vi "String to AUX device cluster.vi"(11 "AUX Device Details":string="GFSF:50:SPD:2:MAN:HVER:1:FVER:0.1:SERL:1837600001:MAN:GMIN:5:TES:3:SIG:OPEN:50.6:STEP:7:SIG:GEAR:6:TVES:19:AUX") -> (3 "Auxiliary Device":T1 {"Signals"."% Open" min=0.0 max=100.0 step=0.1 format="%.4f"; "Signals"."Position" max=20.0 step=1.0 format="%.4f"; "Speed" max=7 step=1; "Gear" max=7 step=1; "Temp V Err" min=0.0 max=20.0 step=0.1; "Temp Err" min=0.0 max=20.0 step=0.1; "Scaling Factor" min=0.0 max=99.0 step=0.1; "Min Flow" min=0.0 max=20.0 step=0.1})   [LabVIEW 2019, in "Mercury iXX.lvlib" / "Auxiliary.lvlib"]
uses:
  Auxiliary.lvlib
  Controls/AUX Device (Read).ctl
  Controls/Manufacturing Data.ctl
  Controls/AUX Signals (Read).ctl
  Mercury iXX.lvlib
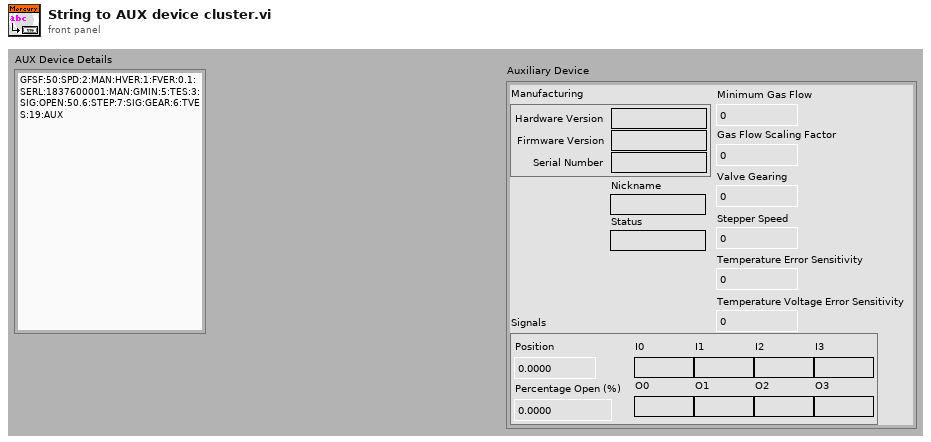
[diagram p1: front panel]
types:
  T1 = typedef "Mercury iXX.lvlib/Auxiliary.lvlib/AUX Device (Read).ctl" = cluster{"Manufacturing":T2, "Min Flow":dbl, "Scaling Factor":dbl, "Temp Err":dbl, "Temp V Err":dbl, "Gear":u32, "Speed":u32, "Signals":T3, "Nickname":string, "Status":string}
  T2 = typedef "Mercury iXX.lvlib/Manufacturing Data.ctl" = cluster{"Hardware Version":string, "Firmware Version":string, "Serial Number":string}
  T3 = typedef "Mercury iXX.lvlib/Auxiliary.lvlib/AUX Signals (Read).ctl" = cluster{"Position":dbl, "% Open":dbl, "I0":string, "I1":string, "I2":string, "I3":string, "O0":string, "O1":string, "O2":string, "O3":string}
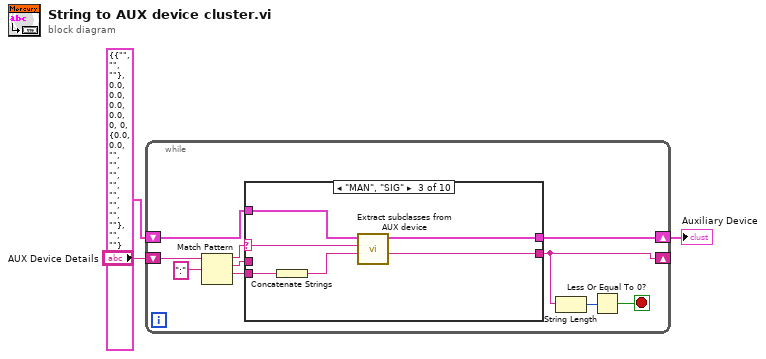
[diagram p0: block diagram]
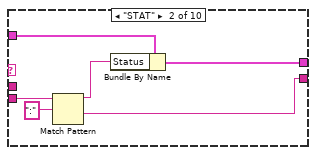
[diagram p3: hidden frame]
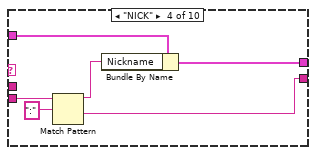
[diagram p4: hidden frame]
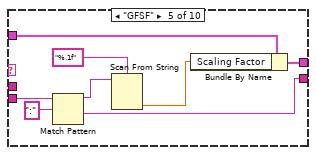
[diagram p5: hidden frame]
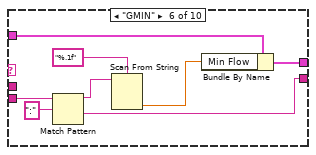
[diagram p6: hidden frame]
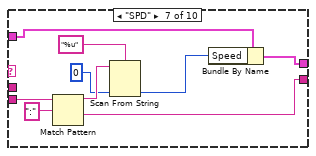
[diagram p7: hidden frame]
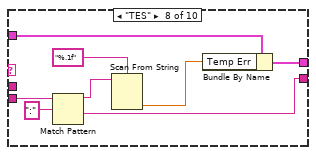
[diagram p8: hidden frame]
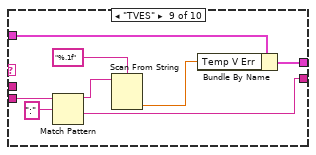
[diagram p9: hidden frame]
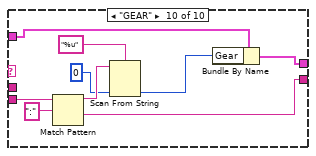
[diagram p10: hidden frame]
diagram:
  n1 = while {
    shift-right: [w9] -> w2
    shift-left: T1 {"Manufacturing"={"Hardware Version"="", "Firmware Version"="", "Serial Number"=""}, "Min Flow"=0.0, "Scaling Factor"=0.0, "Temp Err"=0.0, "Temp V Err"=0.0, "Gear"=0, "Speed"=0, "Signals"={"Position"=0.0, "% Open"=0.0, "I0"="", "I1"="", "I2"="", "I3"="", "O0"="", "O1"="", "O2"="", "O3"=""}, "Nickname"="", "Status"=""} ("Auxiliary Device") -> [w10]
    shift-right: [w5] -> _
    shift-left: "AUX Device Details" -> [w12]
    stop <- w4 stop-if-true
    n2 = Match Pattern(string=w12, regular expression=":") -> (before substring=w11:string, match substring=w8:string, after substring=w7:string)  [unwired: 2 out]
    n3 = case shown="\"MAN\", \"SIG\"" w11 {
      selector: w11 -> [_ _ w27 _ _ _ _ _ _ _]
      tunnel: w8 -> [_ _ _ _ _ _ _ _ _ _]
      tunnel: w10 -> [w15 w18 w22 w30 w39 w47 w56 w64 w72 w81]
      tunnel: [w15 w17 w23 w29 w38 w46 w55 w63 w71 w80] -> w9
      tunnel: [w14 w19 w26 w31 w36 w44 w53 w61 w69 w78] -> w5
      tunnel: w7 -> [w14 w20 w24 w32 w40 w48 w57 w65 w73 w82]
      frame "", Default {
      }
      frame "STAT" {
        n4 = Match Pattern(string=w20, regular expression=":") -> (before substring=w16:string, after substring=w19:string)  [unwired: 3 out]
        n5 = Bundle By Name(cluster=w18, "Status"=w16) -> (w17:T1)
      }
      frame "MAN", "SIG" {
        n6 = Concatenate Strings(w24) -> (w25:string)
        n7 = call "Extract subclasses from AUX device.vi"("Data In"=w25, "Class"=w27, "Aux Device Settings in"=w22) -> ("Data out"=w26:string, "Aux Device Settings out"=w23:T1)  [unwired: 1 in, 6 out]
      }
      frame "NICK" {
        n8 = Match Pattern(string=w32, regular expression=":") -> (before substring=w28:string, after substring=w31:string)  [unwired: 3 out]
        n9 = Bundle By Name(cluster=w30, "Nickname"=w28) -> (w29:T1)
      }
      frame "GFSF" {
        n10 = Match Pattern(string=w40, regular expression=":") -> (before substring=w37:string, after substring=w36:string)  [unwired: 3 out]
        n11 = Scan From String(format string="%.1f", input string=w37) -> (output 1=w35:dbl)  [unwired: 2 in, 4 out]
        n12 = Bundle By Name(cluster=w39, "Scaling Factor"=w35) -> (w38:T1)
      }
      frame "GMIN" {
        n13 = Match Pattern(string=w48, regular expression=":") -> (before substring=w45:string, after substring=w44:string)  [unwired: 3 out]
        n14 = Scan From String(format string="%.1f", input string=w45) -> (output 1=w43:dbl)  [unwired: 2 in, 4 out]
        n15 = Bundle By Name(cluster=w47, "Min Flow"=w43) -> (w46:T1)
      }
      frame "SPD" {
        n16 = Match Pattern(string=w57, regular expression=":") -> (before substring=w54:string, after substring=w53:string)  [unwired: 3 out]
        n17 = Scan From String(format string="%u", input string=w54, default 1=u32 0 ("default value 1")) -> (output 1=w52:u32)  [unwired: 2 in, 3 out]
        n18 = Bundle By Name(cluster=w56, "Speed"=w52) -> (w55:T1)
      }
      frame "TES" {
        n19 = Match Pattern(string=w65, regular expression=":") -> (before substring=w62:string, after substring=w61:string)  [unwired: 3 out]
        n20 = Scan From String(format string="%.1f", input string=w62) -> (output 1=w60:dbl)  [unwired: 2 in, 4 out]
        n21 = Bundle By Name(cluster=w64, "Temp Err"=w60) -> (w63:T1)
      }
      frame "TVES" {
        n22 = Match Pattern(string=w73, regular expression=":") -> (before substring=w70:string, after substring=w69:string)  [unwired: 3 out]
        n23 = Scan From String(format string="%.1f", input string=w70) -> (output 1=w68:dbl)  [unwired: 2 in, 4 out]
        n24 = Bundle By Name(cluster=w72, "Temp V Err"=w68) -> (w71:T1)
      }
      frame "GEAR" {
        n25 = Match Pattern(string=w82, regular expression=":") -> (before substring=w79:string, after substring=w78:string)  [unwired: 3 out]
        n26 = Scan From String(format string="%u", input string=w79, default 1=u32 0 ("default value 1")) -> (output 1=w77:u32)  [unwired: 2 in, 3 out]
        n27 = Bundle By Name(cluster=w81, "Gear"=w77) -> (w80:T1)
      }
    }
    n28 = String Length(string=w5) -> (length=w6:i32)
    n29 = Less Or Equal To 0?(x=w6) -> (x <= 0?=w4:bool)
  }
  "Auxiliary Device" <- w2
